vi "test_libssh2_sftp_close_handle.vi"() -> ()   [LabVIEW 2013, in "libssh2_integration_tests.lvlib"]
uses:
  libssh2_integration_tests.lvlib
  <vilib>/addons/_JKI Toolkits/Caraya/classes/Test/Test.lvclass
  <vilib>/addons/_JKI Toolkits/Caraya/classes/Assert/Assert.lvclass
  libssh2/libssh2.lvlib
panel:
  out "error out":errorcluster
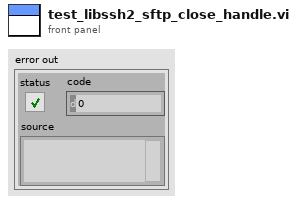
[diagram p1: front panel]
types:
  T1 = typedef "libssh2.lvlib/Session Refnum.ctl" = refnum<k1>
  T2 = typedef "libssh2.lvlib/SFTP Refnum.ctl" = refnum<k1>
  T3 = typedef "libssh2.lvlib/SFTP Handle Refnum.ctl" = refnum<k1>
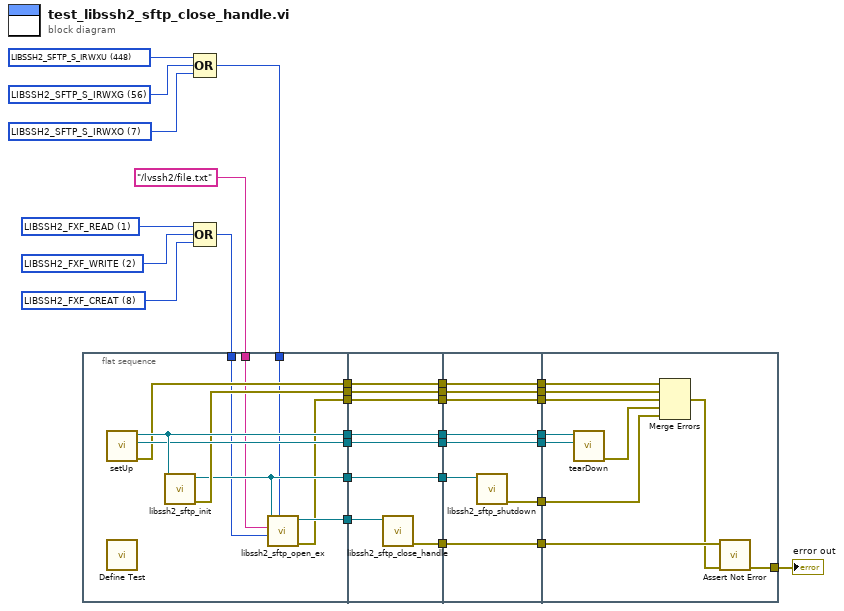
[diagram p0: block diagram]
diagram:
  w24 = u32 2 items=["LIBSSH2_FXF_READ"=1, "LIBSSH2_FXF_WRITE"=2, "LIBSSH2_FXF_APPEND"=4, "LIBSSH2_FXF_CREAT"=8, "LIBSSH2_FXF_TRUNC"=16, "LIBSSH2_FXF_EXCL"=32] ("flags")
  w25 = u32 1 items=["LIBSSH2_FXF_READ"=1, "LIBSSH2_FXF_WRITE"=2, "LIBSSH2_FXF_APPEND"=4, "LIBSSH2_FXF_CREAT"=8, "LIBSSH2_FXF_TRUNC"=16, "LIBSSH2_FXF_EXCL"=32] ("flags")
  w23 = u32 8 items=["LIBSSH2_FXF_READ"=1, "LIBSSH2_FXF_WRITE"=2, "LIBSSH2_FXF_APPEND"=4, "LIBSSH2_FXF_CREAT"=8, "LIBSSH2_FXF_TRUNC"=16, "LIBSSH2_FXF_EXCL"=32] ("flags")
  w28 = 7 items=["LIBSSH2_SFTP_S_IRWXU"=448, "LIBSSH2_SFTP_S_IRUSR"=256, "LIBSSH2_SFTP_S_IWUSR"=128, "LIBSSH2_SFTP_S_IXUSR"=64, "LIBSSH2_SFTP_S_IRWXG"=56, "LIBSSH2_SFTP_S_IRGRP"=32, "LIBSSH2_SFTP_S_IWGRP"=16, "LIBSSH2_SFTP_S_IXGRP"=8, "LIBSSH2_SFTP_S_IRWXO"=7, "LIBSSH2_SFTP_S_IROTH"=4, "LIBSSH2_SFTP_S_IWOTH"=2, "LIBSSH2_SFTP_S_IXOTH"=1] ("mode")
  w29 = 56 items=["LIBSSH2_SFTP_S_IRWXU"=448, "LIBSSH2_SFTP_S_IRUSR"=256, "LIBSSH2_SFTP_S_IWUSR"=128, "LIBSSH2_SFTP_S_IXUSR"=64, "LIBSSH2_SFTP_S_IRWXG"=56, "LIBSSH2_SFTP_S_IRGRP"=32, "LIBSSH2_SFTP_S_IWGRP"=16, "LIBSSH2_SFTP_S_IXGRP"=8, "LIBSSH2_SFTP_S_IRWXO"=7, "LIBSSH2_SFTP_S_IROTH"=4, "LIBSSH2_SFTP_S_IWOTH"=2, "LIBSSH2_SFTP_S_IXOTH"=1] ("mode")
  w30 = 448 items=["LIBSSH2_SFTP_S_IRWXU"=448, "LIBSSH2_SFTP_S_IRUSR"=256, "LIBSSH2_SFTP_S_IWUSR"=128, "LIBSSH2_SFTP_S_IXUSR"=64, "LIBSSH2_SFTP_S_IRWXG"=56, "LIBSSH2_SFTP_S_IRGRP"=32, "LIBSSH2_SFTP_S_IWGRP"=16, "LIBSSH2_SFTP_S_IXGRP"=8, "LIBSSH2_SFTP_S_IRWXO"=7, "LIBSSH2_SFTP_S_IROTH"=4, "LIBSSH2_SFTP_S_IWOTH"=2, "LIBSSH2_SFTP_S_IXOTH"=1] ("mode")
  n1 = flat-sequence {
    tunnel: [w41] -> w15
    tunnel: [w40] -> w13
    tunnel: [w37] -> w11
    tunnel: [w39] -> w8
    tunnel: [w38] -> w6
    tunnel: w27 -> [w36]
    tunnel: "/lvssh2/file.txt" ("filename") -> [w35]
    tunnel: w22 -> [w34]
    tunnel: [w33] -> w4
    tunnel: [w32] -> w3
    tunnel: w15 -> [w49]
    tunnel: [w49] -> w14
    tunnel: w13 -> [w48]
    tunnel: [w48] -> w12
    tunnel: w11 -> [w47]
    tunnel: [w47] -> w10
    tunnel: [w43] -> w9
    tunnel: w8 -> [w46]
    tunnel: [w46] -> w7
    tunnel: w6 -> [w45]
    tunnel: [w45] -> w5
    tunnel: w4 -> [w44]
    tunnel: w3 -> [w42]
    tunnel: [w42] -> w2
    tunnel: w14 -> [w57]
    tunnel: [w57] -> w21
    tunnel: w12 -> [w56]
    tunnel: [w56] -> w20
    tunnel: w10 -> [w52]
    tunnel: w9 -> [w55]
    tunnel: [w55] -> w19
    tunnel: w7 -> [w54]
    tunnel: [w54] -> w18
    tunnel: w5 -> [w53]
    tunnel: [w53] -> w17
    tunnel: [w51] -> w16
    tunnel: w2 -> [w50]
    tunnel: [w50] -> w1
    tunnel: w21 -> [w67]
    tunnel: w20 -> [w66]
    tunnel: w19 -> [w65]
    tunnel: w18 -> [w64]
    tunnel: [w61] -> w31
    tunnel: w17 -> [w60]
    tunnel: w16 -> [w59]
    tunnel: w1 -> [w58]
    frame #0 {
      n2 = call "setUp.vi"() -> ("error out"=w39:errorcluster, "connection ID"=w40:refnum<k5>, "session"=w41:T1)  [unwired: 9 in]
      n3 = call <vilib>:"Define Test.vi"() -> ()  [unwired: 10 in, 2 out]
      n4 = call "libssh2_sftp_init.vi"("session"=w41) -> ("error out"=w38:errorcluster, "sftp"=w37:T2)  [unwired: 9 in]
      n5 = call "libssh2_sftp_open_ex.vi"("mode"=w36, "flags"=w34, "filename"=w35, "sftp"=w37) -> ("error out"=w32:errorcluster, "sftp handle"=w33:T3)  [unwired: 6 in]
    }
    frame #1 {
      n6 = call "libssh2_sftp_close_handle.vi"("sftp handle"=w44) -> ("error out"=w43:errorcluster)  [unwired: 10 in]
    }
    frame #2 {
      n7 = call "libssh2_sftp_shutdown.vi"("sftp"=w52) -> ("error out"=w51:errorcluster)  [unwired: 10 in]
    }
    frame #3 {
      n8 = call "tearDown.vi"("connection ID"=w66, "session"=w67) -> ("error out"=w63:errorcluster)  [unwired: 9 in]
      n9 = Merge Errors(w64, w60, w58, w63, w59) -> (w62:errorcluster)
      n10 = call <vilib>:"Assert Not Error.vi"("error in (no error)"=w62, "Not Error?"=w65) -> ("error out"=w61:errorcluster)  [unwired: 8 in, 1 out]
    }
  }
  n11 = Compound Arithmetic op=OR(w30, w29, w28) -> (w27:i32)
  n12 = Compound Arithmetic op=OR(w25, w24, w23) -> (w22:u32)
  "error out" <- w31
